vi "Global 1.vi"() -> ()   [LabVIEW 2014]
panel:
  out "Servo Angle":dbl
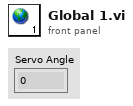
[diagram p1: front panel]
diagram:
